vi "KG get gas ff fn.vi"(8 "Fehler (Eingang, kein Fehler)":errorcluster, 10 "mfc":u32, 11 "VISA-Ressourcenname":refnum<visa-resource-name>) -> (0 "Fehler (Ausgang)":errorcluster, 2 "gasnamen":string[](array[string]), 3 "VISA-Ressourcenname (Ausgang)":refnum<visa-resource-name>, 4 "Kommandos gesendet":string)   [LabVIEW 2020, in "Linearisierung v2.lvlib" / "Gasteiler.lvlib" / "HovaCAL_Interface.lvlib" / "KGN.lvlib" / "get.lvlib"]
uses:
  get.lvlib
  KGN.lvlib
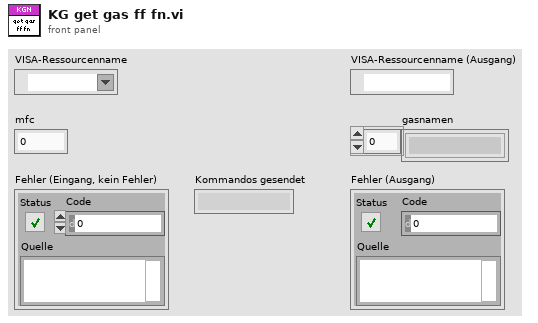
[diagram p1: front panel]
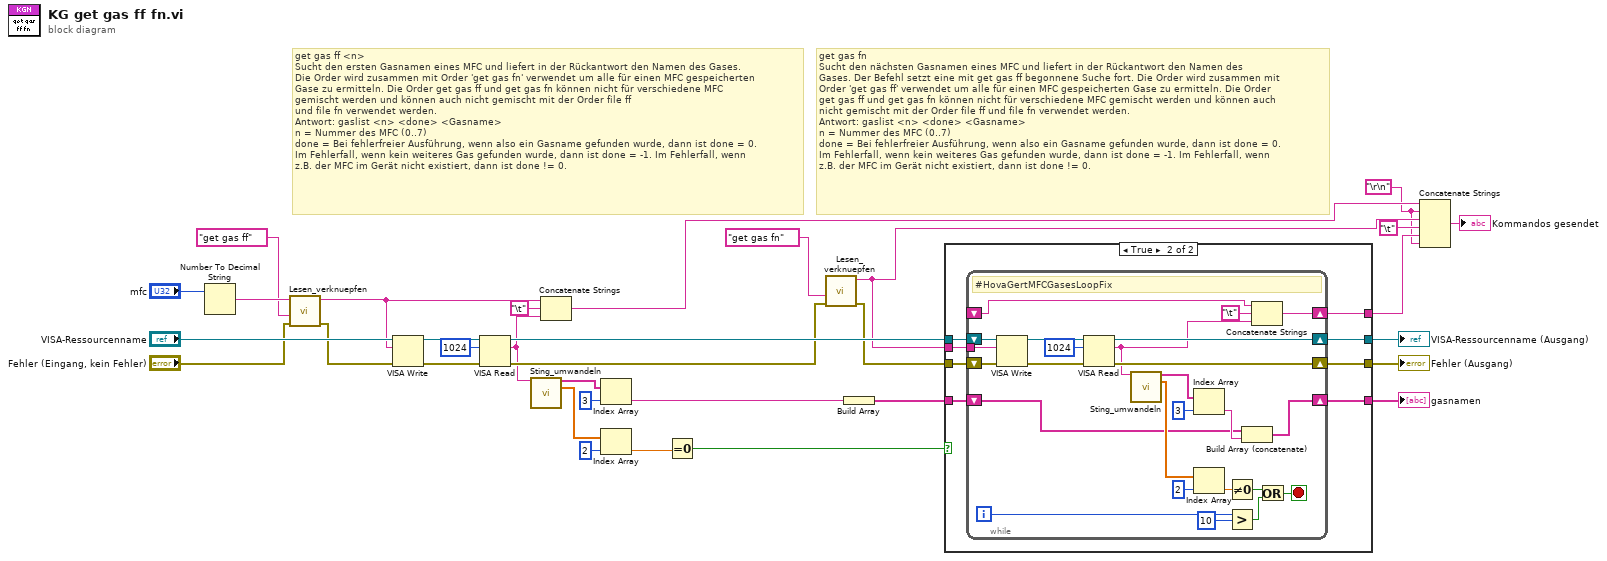
[diagram p0: block diagram]
diagram:
  w2 = "\r\n"
  # "get gas fn\nSucht den nächsten Gasnamen eines MFC und liefert in der Rückantwort den Namen des\nGases. Der Befehl setzt eine mit get gas ff begonnene Suche fort. Die Order wird zusammen mit\nOrder 'get gas ff' verwendet um alle für einen MFC gespeicherten Gase zu ermitteln. Die Order\nget gas ff und get gas fn können nicht für verschiedene MFC gemischt werden und können auch\nnicht gemischt mit der Order file ff und file fn verwendet werden.\nAntwort: gaslist <n> <done> <Gasname>\nn = Nummer des MFC (0..7)\ndone = Bei fehlerfreier Ausführung, wenn also ein Gasname gefunden wurde, dann ist done = 0.\nIm Fehlerfall, wenn kein weiteres Gas gefunden wurde, dann ist done = -1. Im Fehlerfall, wenn\nz.B. der MFC im Gerät nicht existiert, dann ist done != 0."
  # "get gas ff <n>\nSucht den ersten Gasnamen eines MFC und liefert in der Rückantwort den Namen des Gases.\nDie Order wird zusammen mit Order 'get gas fn' verwendet um alle für einen MFC gespeicherten\nGase zu ermitteln. Die Order get gas ff und get gas fn können nicht für verschiedene MFC\ngemischt werden und können auch nicht gemischt mit der Order file ff\nund file fn verwendet werden.\nAntwort: gaslist <n> <done> <Gasname>\nn = Nummer des MFC (0..7)\ndone = Bei fehlerfreier Ausführung, wenn also ein Gasname gefunden wurde, dann ist done = 0.\nIm Fehlerfall, wenn kein weiteres Gas gefunden wurde, dann ist done = -1. Im Fehlerfall, wenn\nz.B. der MFC im Gerät nicht existiert, dann ist done != 0."
  n1 = Number To Decimal String(number="mfc") -> (decimal integer string=w26:string)  [unwired: 1 in]
  n2 = call "Lesen_verknuepfen.vi"("error in (no error)"="Fehler (Eingang, kein Fehler)", "Order"="get gas ff" ("Schreibpuffer"), "param"=w26) -> ("error out"=w27:errorcluster, "Verknüpfter String"=w9:string)  [unwired: 7 in]
  n3 = VISA Write(VISA resource name="VISA-Ressourcenname", write buffer=w9, error in (no error)=w27) -> (VISA resource name out=w33:refnum<visa-resource-name>, error out=w32:errorcluster)  [unwired: 1 out]
  n4 = VISA Read(VISA resource name=w33, byte count=u32 1024 ("Byte-Anzahl"), error in (no error)=w32) -> (VISA resource name out=w19:refnum<visa-resource-name>, read buffer=w8:string, error out=w15:errorcluster)  [unwired: 1 out]
  n5 = call "Sting_umwandeln.vi"("Lesepuffer"=w8) -> ("string array"=w23:string[], "Zahl array"=w21:dbl[])  [unwired: 8 in, 5 out]
  n6 = Concatenate Strings(w9, "\t", w8) -> (w6:string)
  n7 = Index Array(array=w23, index=3 ("Index")) -> (element=w12:string)
  n8 = Index Array(array=w21, index=2 ("Index")) -> (element=w20:dbl)
  n9 = Equal To 0?(x=w20) -> (x = 0?=w13:bool)
  n10 = call "Lesen_verknuepfen.vi"("error in (no error)"=w15, "Order"="get gas fn" ("Schreibpuffer")) -> ("error out"=w14:errorcluster, "Verknüpfter String"=w5:string)  [unwired: 8 in]
  n11 = Build Array(w12) -> (w11:string[])
  n12 = case shown="True" w13 {
    tunnel: w19 -> [w36 w44]
    tunnel: [w36 w43] -> w18
    tunnel: [w35 w42] -> w17
    tunnel: w5 -> [_ w41]
    tunnel: w14 -> [w35 w40]
    tunnel: w11 -> [w34 w39]
    tunnel: [w34 w38] -> w10
    tunnel: [_ w37] -> w3
    frame False {
    }
    frame True {
      n13 = while {
        tunnel: w41 -> [w63]
        shift-right: [w65] -> w43
        shift-left: w44 -> [w66]
        shift-right: [w64] -> w42
        shift-left: w40 -> [w62]
        shift-right: [w53] -> w38
        shift-left: w39 -> [w54]
        shift-right: [w46] -> w37
        shift-left: _ -> [w45]
        i -> [w50]
        stop <- w52 stop-if-true
        # "#HovaGertMFCGasesLoopFix"
        n14 = VISA Write(VISA resource name=w66, write buffer=w63, error in (no error)=w62) -> (VISA resource name out=w67:refnum<visa-resource-name>, error out=w68:errorcluster)  [unwired: 1 out]
        n15 = VISA Read(VISA resource name=w67, byte count=u32 1024 ("Byte-Anzahl"), error in (no error)=w68) -> (VISA resource name out=w65:refnum<visa-resource-name>, read buffer=w47:string, error out=w64:errorcluster)  [unwired: 1 out]
        n16 = call "Sting_umwandeln.vi"("Lesepuffer"=w47) -> ("string array"=w56:string[], "Zahl array"=w60:dbl[])  [unwired: 8 in, 5 out]
        n17 = Index Array(array=w56, index=3 ("Index")) -> (element=w55:string)
        n18 = Index Array(array=w60, index=2 ("Index")) -> (element=w58:dbl)
        n19 = Not Equal To 0?(x=w58) -> (x != 0?=w59:bool)
        n20 = Greater?(x=w50, y=10) -> (0:w51:bool)
        n21 = Build Array (concatenate)(w54, w55) -> (w53:string[])
        n22 = Concatenate Strings(w45, "\t", w47) -> (w46:string)
        n23 = Or(x=w59, y=w51) -> (x .or. y?=w52:bool)
      }
    }
  }
  "VISA-Ressourcenname (Ausgang)" <- w18
  "Fehler (Ausgang)" <- w17
  "gasnamen" <- w10
  n24 = Concatenate Strings(w6, w2, w5, "\t", w3, w2) -> (→"Kommandos gesendet":string)
